vi "FPGA_TDCexperiment.vi"() -> ()   [LabVIEW 2017]
uses:
  RSNRPZ/RSNRPZcontrol.ctl
  <vilib>/FPGAPlugInAG/PXI-7842R/niLvFpga_Open_PXI-7842R.vi
  <vilib>/rvi/interface/common/dynamic/niFpgaDynamicAddResources.vi
  <vilib>/Utility/error.llb/Error Cluster From Error Code.vi
  <vilib>/rvi/errors/niLvFpgaAdjustHostInterfaceError.vi
  <vilib>/rvi/interface/common/niFpgaWaitOnOcc.vi
  <vilib>/FPGAPlugInAG/Dynamic/niLvFpga_Close_Dynamic.vi
  <vilib>/rvi/interface/nirviOpenFPGA/nirviOpenFPGA.xnode
  FPGA_bitfile/Jarvis_FPGATargetMacro_281119TDCLV2017_HUsPPJBlkv4.lvbitx
  <vilib>/rvi/interface/nirviReadWriteControl/nirviReadWriteControl.xnode
  <vilib>/rvi/interface/nirviMethod/nirviMethod.xnode
  <vilib>/rvi/interface/nirviCloseFPGA/nirviCloseFPGA.xnode
  NiFpgaLv.dll
  <vilib>/rvi/interface/Simulation/niFpgaSimulationCallBeginRW.vi
  <vilib>/FPGAPlugInAG/Dynamic/niLvFpga_ConfigureFifo_Dynamic.vi
  <vilib>/rvi/errors/niLvFpgaMergeErrorWithErrorCode.vi
  <vilib>/FPGAPlugInAG/Dynamic/niLvFpga_ReadFifo_Dynamic.vi
panel:
  out "Histogram":dynamicdata(graph)
  in  "N photons":u32=20
  out "Waveform Chart":u32[](graph)
  in  "runTDC":bool=TRUE
  in  "stop":bool
  in  "RSNPRZsettings":T1={"Average Counts :"=1.0, "Correction Freq [MHz] :"=50.0, "Integration Time [ms] : "=0.1, "P :"=0.0, "I :"=0.0, "D :"=0.0, "Power setpoint :"=0.0, "PID on :"=FALSE, "Voltage :"=0.0, "Reset :"=FALSE, "Agilient Power Level [dBm] :"=0.0} caption="RSNPRZ Settings :" {"Agilient Power Level [dBm] :" format="%_3g"; "Voltage :" format="%_5g"; "Power setpoint :" format="%_4g"; "D :" format="%_4g"; "I :" format="%_4g"; "P :" format="%_4g"; "Integration Time [ms] :" format="%_3g"; "Correction Freq [MHz] :" format="%_4g"}
  out "FPGAerr":bool=TRUE
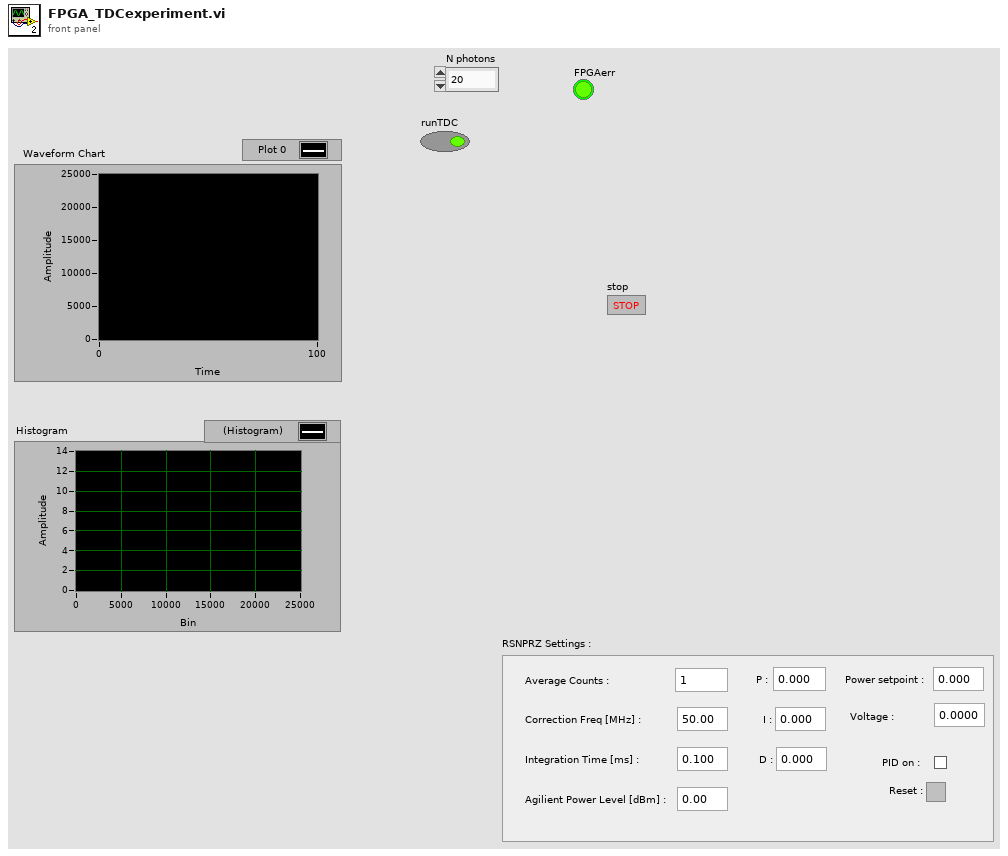
[diagram p1: front panel]
types:
  T1 = typedef "RSNRPZcontrol.ctl" = cluster{"Average Counts :":dbl, "Correction Freq [MHz] :":dbl, "Integration Time [ms] : ":dbl, "P :":dbl, "I :":dbl, "D :":dbl, "Power setpoint :":dbl, "PID on :":bool, "Voltage :":dbl, "Reset :":bool, "Agilient Power Level [dBm] :":dbl}
  T2 = cluster{"HighPowerNum":dbl, "LowPowerNum":dbl, "PIDnum":dbl, "DeltaFreq":dbl, "BaseFreq":dbl, "AOMout":dbl, "ButtonSelected":enum16{"PID", "Low", "High"}, "AO3":bool}
  T3 = cluster{"DIO 0":bool, "DIO 1":bool, "DIO 2":bool, "DIO 3":bool, "DIO 4":bool, "DIO 5":bool, "DIO 6":bool, "DIO 7":bool, "DIO 8":bool, "DIO 9":bool, "DIO 10":bool, "DIO 11":bool, "DIO 12":bool, "DIO 13":bool, "DIO 14":bool, "DIO 15":bool, "DIO 16":bool, "DIO 17":bool, "DIO 18":bool, "DIO 19":bool, "DIO 20":bool, "DIO 21":bool, "DIO 22":bool, "DIO 23":bool, "DIO 24":bool, "DIO 25":bool, "DIO 26":bool, "DIO 27":bool, "DIO 28":bool, "DIO 29":bool, "DIO 30":bool, "DIO 31":bool, "DIO 32":bool, "DIO 33":bool, "DIO 34":bool, "DIO 35":bool, "DIO 36":bool, "DIO 37":bool, "DIO 38":bool, "DIO 39":bool}
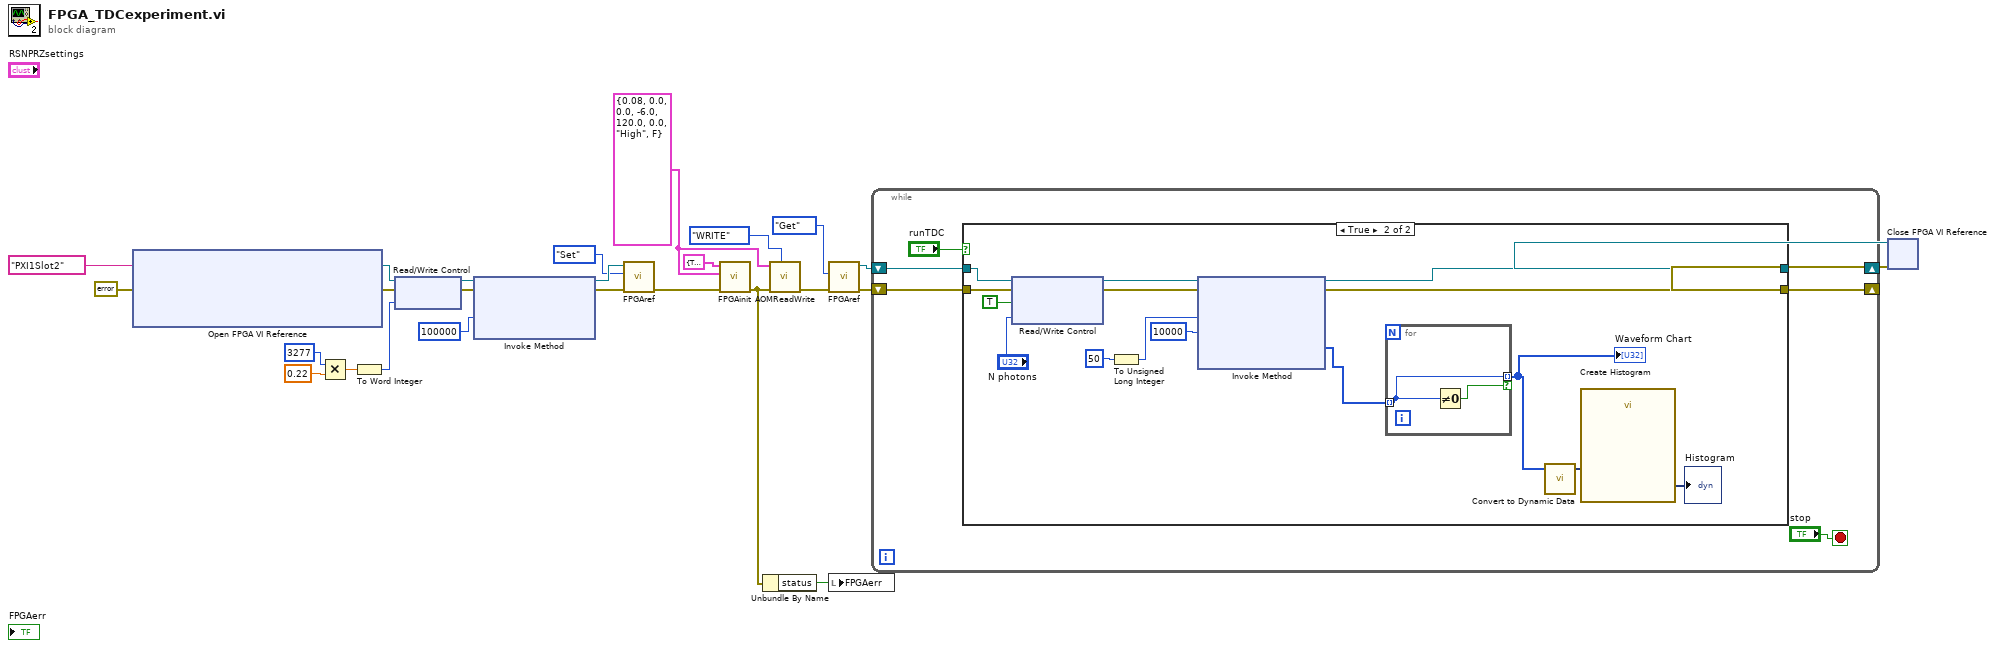
[diagram p0: block diagram]
diagram:
  w3 = T2 {"HighPowerNum"=0.08, "LowPowerNum"=0.0, "PIDnum"=0.0, "DeltaFreq"=-6.0, "BaseFreq"=120.0, "AOMout"=0.0, "ButtonSelected"=enum."High", "AO3"=FALSE} ("AOMsetting")
  n1 = xnode "Open FPGA VI Reference"("error in"=errorcluster {"status"=FALSE, "code"=0, "source"=""}, "resource name"=tag "PXI1Slot2") -> ("FPGA VI Reference Out"=w19:refnum<k20>, "error out"=w17:errorcluster)
  n2 = Multiply(x=3277, y=0.22) -> (x*y=w13:dbl)
  n3 = To Word Integer(number=w13) -> (16bit integer=w12:i16)
  n4 = xnode "Read/Write Control"("FPGA VI Reference In"=w19, "error in"=w17, "AO4 max"=w12) -> ("FPGA VI Reference Out"=w18:refnum<k20>, "error out"=w16:errorcluster)
  n5 = xnode "Invoke Method"("FPGA VI Reference In"=w18, "error in"=w16, "Requested Depth"=u32 100000) -> ("FPGA VI Reference Out"=w24:refnum<k20>, "error out"=w25:errorcluster)  [unwired: 1 out]
  n6 = call "FPGAref.vi"("error in"=w25, "Enum"=enum16{"Set", "Get"}."Set", "FPGA VI Reference Out"=w24) -> ("error out"=w22:errorcluster)  [unwired: 3 in, 1 out]
  n7 = call "FPGAinit.vi"("error in"=w22, "XAOMsetting"=w3, "DIOcluster"=T3 {"DIO 0"=TRUE, "DIO 1"=FALSE, "DIO 2"=FALSE, "DIO 3"=FALSE, "DIO 4"=FALSE, "DIO 5"=FALSE, "DIO 6"=FALSE, "DIO 7"=FALSE, "DIO 8"=FALSE, "DIO 9"=FALSE, "DIO 10"=FALSE, "DIO 11"=FALSE, "DIO 12"=TRUE, "DIO 13"=FALSE, "DIO 14"=FALSE, "DIO 15"=FALSE, "DIO 16"=FALSE, "DIO 17"=TRUE, "DIO 18"=FALSE, "DIO 19"=FALSE, "DIO 20"=FALSE, "DIO 21"=FALSE, "DIO 22"=FALSE, "DIO 23"=FALSE, "DIO 24"=FALSE, "DIO 25"=FALSE, "DIO 26"=FALSE, "DIO 27"=FALSE, "DIO 28"=FALSE, "DIO 29"=FALSE, "DIO 30"=FALSE, "DIO 31"=FALSE, "DIO 32"=FALSE, "DIO 33"=FALSE, "DIO 34"=FALSE, "DIO 35"=FALSE, "DIO 36"=FALSE, "DIO 37"=FALSE, "DIO 38"=FALSE, "DIO 39"=FALSE}) -> ("error out"=w10:errorcluster)  [unwired: 8 in]
  n8 = Unbundle By Name(w10) -> ("status"=w21:bool)
  n9 = call "AOMReadWrite.vi"("Enum"=enum16{"READ", "WRITE"}."WRITE", "error in"=w10, "XAOMsetting"=w3) -> ("error out"=w9:errorcluster)  [unwired: 6 in, 2 out]
  n10 = call "FPGAref.vi"("error in"=w9, "Enum"=enum16{"Set", "Get"}."Get") -> ("error out"=w5:errorcluster, "FPGA VI Reference Out 2"=w2:refnum<k20>)  [unwired: 4 in]
  n11 = local write "FPGAerr"(w21) -> ()
  n12 = while {
    shift-right: [w29] -> w1
    shift-left: w2 -> [w30]
    shift-right: [w28] -> w6
    shift-left: w5 -> [w27]
    stop <- "stop" stop-if-true
    n13 = case shown="True" "runTDC" {
      tunnel: w30 -> [w34 w47]
      tunnel: [w34 w41] -> w29
      tunnel: [w33 w40] -> w28
      tunnel: w27 -> [w33 w39]
      frame False {
      }
      frame True {
        n14 = xnode "Read/Write Control"("FPGA VI Reference In"=w47, "error in"=w39, "Acquire times"=TRUE, "N photons"="N photons") -> ("FPGA VI Reference Out"=w43:refnum<k20>, "error out"=w42:errorcluster)
        n15 = To Unsigned Long Integer(number=50) -> (unsigned 32bit integer=w44:u32)
        n16 = xnode "Invoke Method"("FPGA VI Reference In"=w43, "error in"=w42, "Number of Elements"=w44, "Timeout (ms)"=10000) -> ("FPGA VI Reference Out"=w41:refnum<k20>, "error out"=w40:errorcluster, "Data"=w38:u32[])  [unwired: 1 out]
        n17 = for {
          tunnel: w38 -> [w51] mode=indexing
          tunnel: [w51] -> w35 mode=indexing if=w50
          n18 = Not Equal To 0?(x=w51) -> (x != 0?=w50:bool)
        }
        "Waveform Chart" <- w35
        n19 = call "Convert to Dynamic Data"("Array"=w35) -> ("Dynamic Data Type"=w36:dynamicdata)  [unwired: 3 in]
        n20 = call "Create Histogram"("Signal"=w36) -> ("Histogram"=→"Histogram":dynamicdata)  [unwired: 9 in, 1 out]
      }
    }
  }
  n21 = xnode "Close FPGA VI Reference"("FPGA VI Reference In"=w1, "error in"=w6) -> ()  [unwired: 1 out]
